vi "NI VeriStand - Search for Item by GUID.vi"(7 "Direction (Down)":T1, 8 "error in":errorcluster, 10 "Item GUID":string, 11 "Section Ref in":T2 format="%.0x") -> (0 "error out":errorcluster, 2 "Item Ref":T2 format="%.0x", 3 "Section Ref out":T2 format="%.0x", 4 "Found":bool)   [LabVIEW 2020, in "Custom Device Utility Library.lvlib"]
doc: "Searches a custom device section for the item(s) you specify. You can search for one or multiple items by name, GUID, or property name and value. You must manually select the polymorphic instance to use."
uses:
  <vilib>/NI VeriStand/Custom Device Tools/Custom Device Utility Library/Custom Device Utility Library.lvlib
  <vilib>/NI VeriStand/Custom Device API/Custom Device Item Ref.ctl
  <vilib>/NI VeriStand/Custom Device Tools/Custom Device Utility Library/Search Direction.ctl
  <vilib>/NI VeriStand/Custom Device Tools/Custom Device Utility Library/NI VeriStand - Ref Constants.vi
  <vilib>/NI VeriStand/Custom Device API/Custom Device API.lvlib
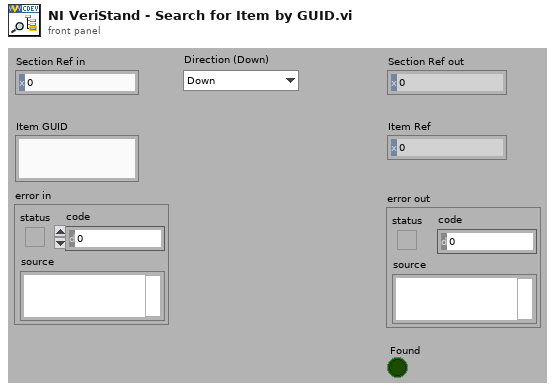
[diagram p1: front panel]
types:
  T1 = typedef "Custom Device Utility Library.lvlib/Search Direction.ctl" = enum16{"Down", "Up"}
  T2 = typedef "Custom Device API.lvlib/Custom Device Item Ref.ctl" = u64
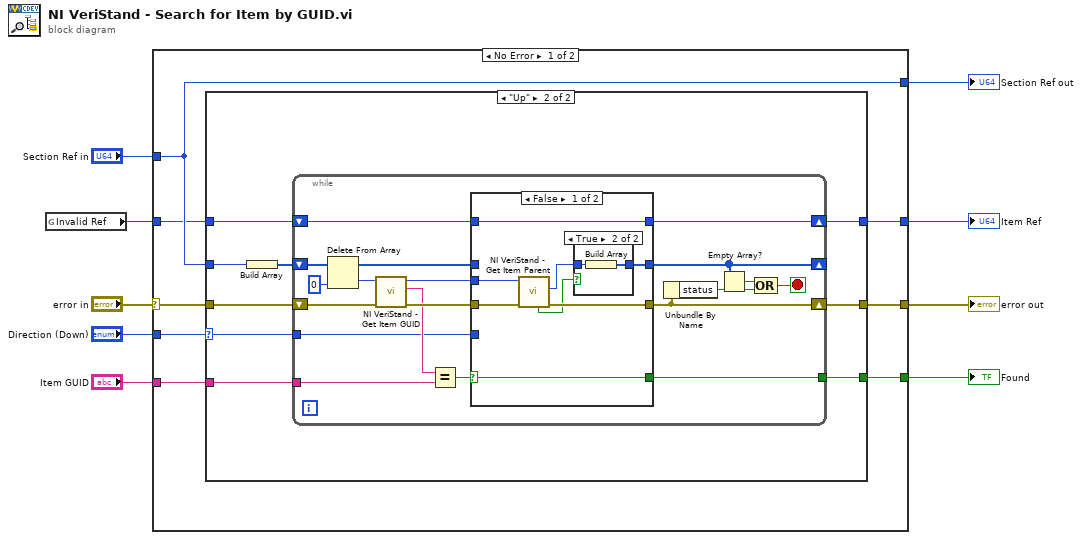
[diagram p0: block diagram]
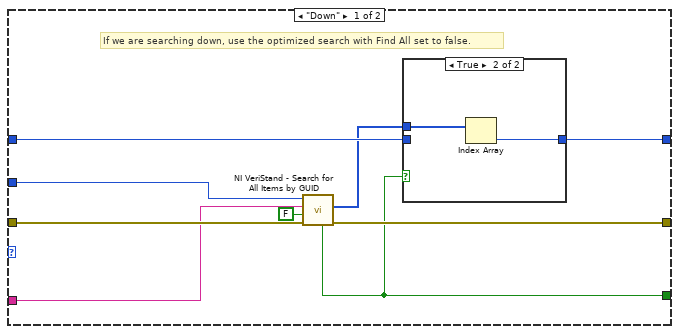
[diagram p2: hidden frame]
diagram:
  n1 = global read "NI VeriStand - Ref Constants.vi" "Invalid Ref"() -> (w2:T2)
  n2 = case shown="No Error" "error in" {
    selector: "error in" -> [w13 w72]
    tunnel: "Section Ref in" -> [w14 w73]
    tunnel: "Item GUID" -> [w17 _]
    tunnel: [w16 w72] -> w7
    tunnel: [w15 _] -> w6
    tunnel: [w12 w71] -> w5
    tunnel: [w14 w73] -> w4
    tunnel: w2 -> [w11 w71]
    tunnel: "Direction (Down)" -> [w10 _]
    frame No Error {
      n3 = case shown="\"Up\"" w10 {
        selector: w10 -> [_ w30]
        tunnel: w17 -> [w23 w37]
        tunnel: [w24 w36] -> w16
        tunnel: [w20 w35] -> w15
        tunnel: w14 -> [w26 w34]
        tunnel: w13 -> [w25 w33]
        tunnel: [w22 w32] -> w12
        tunnel: w11 -> [w19 w31]
        frame "Down" {
          # "If we are searching down, use the optimized search with Find All set to false."
          n4 = call <vilib>:"NI VeriStand - Search for All Items by GUID.vi"("error in"=w25, "Find All? (T)"=FALSE, "Item GUID"=w23, "Section Ref in"=w26) -> ("error out"=w24:errorcluster, "Item Refs"=w18:T2[], "Found"=w20:bool)  [unwired: 4 in, 1 out]
          n5 = case shown="True" w20 {
            tunnel: w18 -> [_ w29]
            tunnel: [w27 w28] -> w22
            tunnel: w19 -> [w27 _]
            frame False {
            }
            frame True {
              n6 = Index Array(array=w29) -> (element=w28:T2)  [unwired: 1 in]
            }
          }
        }
        frame "Up" {
          n7 = Build Array(w34) -> (w38:T2[])
          n8 = while {
            shift-right: [w42] -> w36
            shift-left: w33 -> [w56]
            shift-right: [w41] -> _
            shift-left: w38 -> [w55]
            tunnel: w37 -> [w52]
            tunnel: [w47] -> w35
            shift-right: [w49] -> w32
            shift-left: w31 -> [w46]
            tunnel: w30 -> [w40]
            stop <- w43 stop-if-true
            n9 = Delete From Array(array=w55, index=0) -> (deleted portion=w39:T2, array with subset deleted=w50:T2[])  [unwired: 1 in]
            n10 = call <vilib>:"NI VeriStand - Get Item GUID.vi"("error in (no error)"=w56, "Item Ref in"=w39) -> ("error out"=w57:errorcluster, "GUID"=w53:string, "Item Ref out"=w51:T2)  [unwired: 7 out]
            n11 = Equal?(x=w53, y=w52) -> (x = y?=w48:bool)
            n12 = case shown="False" w48 {
              selector: w48 -> [w61 w69]
              tunnel: [w65 w70] -> w42
              tunnel: w57 -> [w64 w70]
              tunnel: w51 -> [w63 w68]
              tunnel: w50 -> [_ _]
              tunnel: [w62 _] -> w41
              tunnel: [w60 w68] -> w49
              tunnel: [w61 w69] -> w47
              tunnel: w46 -> [w60 _]
              tunnel: w40 -> [_ _]
              frame False {
                n13 = call <vilib>:"NI VeriStand - Get Item Parent.vi"("error in (no error)"=w64, "Item Ref in"=w63) -> ("error out"=w65:errorcluster, "Parent Ref"=w59:T2, "Found"=w58:bool)  [unwired: 6 in, 1 out]
                n14 = case shown="True" w58 {
                  tunnel: w59 -> [_ w67]
                  tunnel: [_ w66] -> w62
                  frame False {
                  }
                  frame True {
                    n15 = Build Array(w67) -> (w66:T2[])
                  }
                }
              }
              frame True {
              }
            }
            n16 = Unbundle By Name(w42) -> ("status"=w44:bool)
            n17 = Empty Array?(array=w41) -> (empty?=w45:bool)
            n18 = Compound Arithmetic op=OR(w45, w44) -> (w43:bool)
          }
        }
      }
    }
    frame Error {
    }
  }
  "Found" <- w6
  "error out" <- w7
  "Section Ref out" <- w4
  "Item Ref" <- w5
